vi "Curtin1_Share.vi"(11 "Files":T2(array[cluster])) -> ()   [LabVIEW 2022 SP3]
panel:
  in  "Show Notes":bool
  in  "Selections":T1
  # "What do you want to share?"
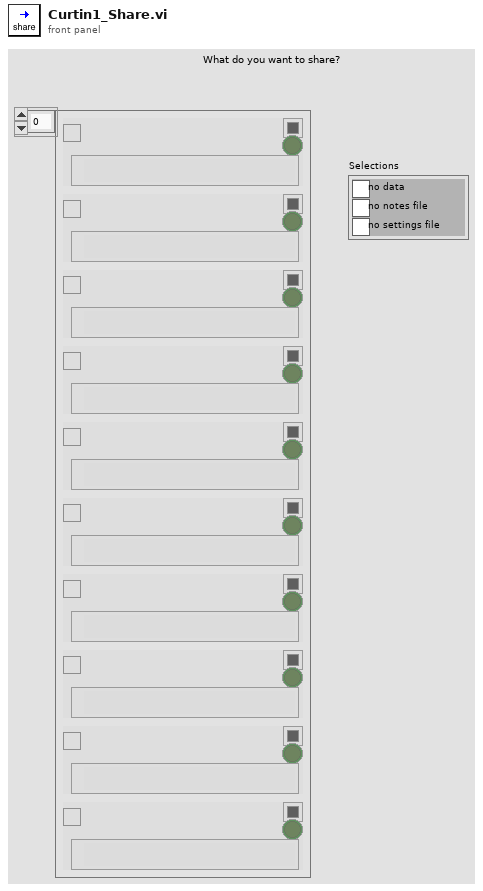
[diagram p1: front panel]
types:
  T1 = cluster{"data":bool, "notes":bool, "settings file":bool}
  T2 = cluster{"Show?":bool, "Name":string, "Color":u32, "Path":path, "Show Notes":bool, "correlate":bool}[]
  T3 = cluster{"Test":string, "Set":string, "Position":string, "Tap":string}
  T4 = cluster{"Show?":bool, "Name":string, "Color":u32, "Path":path, "Show Notes":bool, "correlate":bool}
  T5 = cluster{"Name of test":string, "Date":timestamp, "Location":string, "Template":string, "Soundcard":string, "resolution":u16, "Sampling rate":u16, "Ch1 Gain ":dbl, "Ch2 Gain":dbl, "Sample time (s)":dbl, "Pre-trigger (s)":dbl, "Hammer Threshold":dbl, "Positions":i16, "Taps/Position":i16, "Set Names":string, "Freq resolution":dbl, "Hammer cutoff":dbl, "Mic cutoff":dbl, "Double bounce ":dbl, "Hammer Cal":dbl, "dB Offset":dbl, "Accel Cal":dbl, "Vibrometer Cal":dbl, "Mic Cal":dbl, "Output":u16, "Voltage Cal":dbl, "Vibrometer Port":string, "Range":u16, "High Pass":u16, "Bandwidth":u16, "X Range":cluster{"Minimum":dbl, "Maximum":dbl, "Increment":dbl, "Minor Increment":dbl, "Start":dbl}[], "Y Range":cluster{"Minimum":dbl, "Maximum":dbl, "Increment":dbl, "Minor Increment":dbl, "Start":dbl}[], "dB Spread":dbl, "Trigger":u16, "Ch_1":u8, "Ch_2":u8, "flip?":bool, "60Hz":bool, "Time offset":dbl, "Piezo Cal":dbl, "Default Notes":string, "Tom":bool}
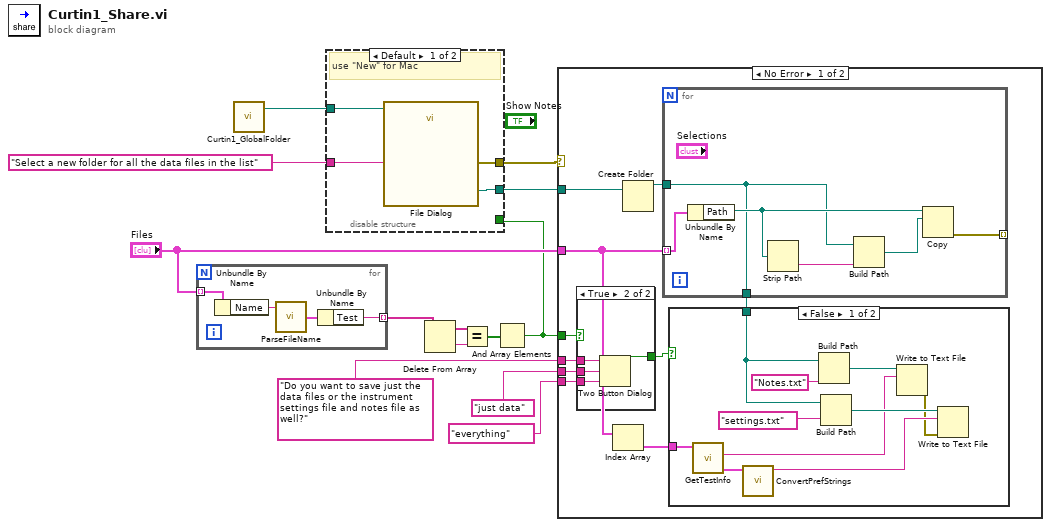
[diagram p0: block diagram]
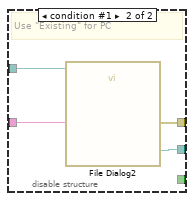
[diagram p2: hidden frame]
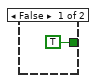
[diagram p4: hidden frame]
diagram:
  n1 = for {
    tunnel: "Files" -> [w17] mode=indexing
    tunnel: [w14] -> w8 mode=indexing
    n2 = Unbundle By Name(w17) -> ("Name"=w16:string)
    n3 = call "ParseFileName.vi"("String in"=w16) -> ("Name"=w15:T3)  [unwired: 2 out]
    n4 = Unbundle By Name(w15) -> ("Test"=w14:string)
  }
  n5 = call "Curtin1_GlobalFolder.vi"() -> ("LabVIEW Data Path"=w10:path)  [unwired: 1 in, 1 out]
  n6 = Delete From Array(array=w8) -> (deleted portion=w6:string, array with subset deleted=w7:string[])  [unwired: 2 in]
  n7 = Equal?(x=w7, y=w6) -> (x = y?=w5:bool[])
  n8 = And Array Elements(Boolean array=w5) -> (logical AND=w1:bool)
  n9 = disable-structure shown="Default" {
    disable-tunnel: [w21 w25] -> w13
    disable-tunnel: "Select a new folder for all the data files in the list" ("prompt") -> [w20 w24]
    disable-tunnel: [w19 w23] -> w11
    disable-tunnel: w10 -> [w18 w22]
    disable-tunnel: w1 -> [_ _]
    frame condition #0 (active) {
      # "use \"New\" for Mac"
      n10 = call "File Dialog"("start path"=w18, "prompt"=w20) -> ("selected path"=w21:path, "error out"=w19:errorcluster)  [unwired: 10 in, 2 out]
    }
    frame condition #1 {
      # "Use \"Existing\" for PC"
      n11 = call "File Dialog2"("start path"=w22, "prompt"=w24) -> ("selected path"=w25:path, "error out"=w23:errorcluster)  [unwired: 10 in, 2 out]
    }
  }
  n12 = case shown="No Error" w11 {
    tunnel: "Files" -> [w28 _]
    tunnel: w13 -> [w35 _]
    tunnel: w1 -> [w33 _]
    tunnel: "Do you want to save just the data files or the instrument settings file and notes file as well?" ("prompt") -> [w32 _]
    tunnel: "just data" ("prompt") -> [w31 _]
    tunnel: "everything" ("prompt") -> [w30 _]
    frame No Error {
      n13 = case shown="True" w33 {
        tunnel: w32 -> [_ w50]
        tunnel: w31 -> [_ w49]
        tunnel: w30 -> [_ w48]
        tunnel: [TRUE ("T button?") w47] -> w29
        frame False {
        }
        frame True {
          n14 = Two Button Dialog(message=w50, 1:w48, 2:w49) -> (T button?=w47:bool)
        }
      }
      n15 = Index Array(array=w28) -> (element=w27:T4)  [unwired: 1 in]
      n16 = Create Folder(path (use dialog)=w35) -> (created path=w34:path)  [unwired: 2 in, 2 out]
      n17 = for {
        tunnel: w28 -> [w56] mode=indexing
        tunnel: w34 -> [w51]
        tunnel: [w52] -> _ mode=indexing
        tunnel: [w51] -> w26
        n18 = Unbundle By Name(w56) -> ("Path"=w55:path)
        n19 = Strip Path(path=w55) -> (name=w54:string)  [unwired: 1 out]
        n20 = Build Path(base path=w51, name or relative path=w54) -> (appended path=w53:path)
        n21 = Copy(10:w53, 11:w55) -> (0:w52:errorcluster)  [unwired: 3 in, 2 out]
      }
      n22 = case shown="False" w29 {
        tunnel: w27 -> [w45 _]
        tunnel: w26 -> [w40 _]
        frame False {
          n23 = call "GetTestInfo.vi"("File selected"=w45) -> ("Settings"=w44:T5, "Notes"=w37:string)  [unwired: 3 in, 6 out]
          n24 = call "ConvertPrefStrings.vi"("Settings"=w44) -> ("String Out"=w43:string)  [unwired: 9 in, 1 out]
          n25 = Build Path(base path=w40, name or relative path="Notes.txt") -> (appended path=w38:path)
          n26 = Build Path(base path=w40, name or relative path="settings.txt" ("prompt")) -> (appended path=w41:path)
          n27 = Write to Text File(file (use dialog)=w38, text=w37) -> (error out=w36:errorcluster)  [unwired: 2 in, 2 out]
          n28 = Write to Text File(file (use dialog)=w41, text=w43, error in=w36) -> ()  [unwired: 1 in, 3 out]
        }
        frame True {
        }
      }
    }
    frame Error {
    }
  }
